vi "GetStatus.vi"(8 "error in (no error)":errorcluster, 11 "S4GUI in":refnum<class "S4GUI.lvclass">) -> (0 "error out":errorcluster, 3 "S4GUI out":refnum<class "S4GUI.lvclass">)   [LabVIEW 2018, in "S4GUI.lvclass"]
uses:
  S4GUI.lvclass
  S4GUI.lvclass/S4GUI.ctl
  Server/Server.lvclass/Server.ctl
  Instrument/Instrument.lvclass/Instrument.ctl
  Device/Optics/Optics.lvclass/Optics.ctl
  Interface/Interface.lvclass/Interface.ctl
  TelFocus/TelFocus.lvclass
  C:/Users/devstaff/sparc4/s4gui/Versao ZeroMQ REQ-REP/SPARC4_GUI -v1.0.0/Server/Server.lvclass
  WeatherStation/WeatherStation.lvclass
  Instrument/Instrument.lvclass
  TCS/TCS.lvclass
  SyncBox/Sync Box.lvclass
  Device/Optics/Opt_Selector/Opt_Selector.lvclass
  C:/Users/devstaff/sparc4/s4gui/Versao ZeroMQ REQ-REP/SPARC4_GUI -v1.0.0/Device/Optics/Optics.lvclass
  Device/Optics/Opt_Continuous/Opt_Continuous.lvclass
  Acquisition/Acquisition.lvclass
  GSserver/GSserver.lvclass
  Channel/Channel.lvclass
  Interface/Interface.lvclass
  GSstatus/GSstatus.lvclass
  SecMirror/SecMirror.lvclass
  WeatherSensor/WeatherSensor.lvclass
  Trigger/Trigger.lvclass
  Device/Optics/Optics.lvclass
  Server/Server.lvclass
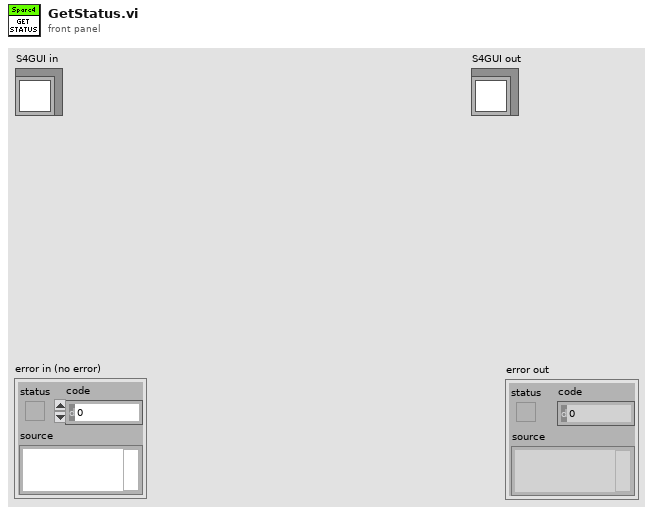
[diagram p1: front panel]
types:
  T1 = cluster{"ACQUISITION_MODE":bool, "TRIGGER_MODE":bool, "READ_MODE":bool, "PREAMP":bool, "READOUT_RATE":bool, "VERTICAL_SHIFT_SPEED":bool, "EM_MODE":bool, "EM_GAIN":bool, "SHUTTER_MODE":bool, "SHUTTER_TTL":bool, "SHUTTER_OPENING_TIME":bool, "SHUTTER_CLOSING_TIME":bool, "VBIN":bool, "HBIN":bool, "INITIAL_LINE":bool, "INITIAL_COLUMN":bool, "FINAL_LINE":bool, "FINAL_COLUMN":bool, "FRAME_TRANSFER":bool, "VERTICAL_CLOCK_VOLTAGE":bool, "AD_CHANNEL":bool}
  T2 = cluster{"ACQUISITION_MODE":u8, "TRIGGER_MODE":u8, "READ_MODE":u8, "PREAMP":u8, "READOUT_RATE":u8, "VERTICAL_SHIFT_SPEED":u8, "EM_MODE":u8, "EM_GAIN":u16, "SHUTTER_MODE":u8, "SHUTTER_TTL":u8, "SHUTTER_OPENING_TIME":u16, "SHUTTER_CLOSING_TIME":u16, "VBIN":u16, "HBIN":u16, "INITIAL_LINE":u16, "INITIAL_COLUMN":u16, "FINAL_LINE":u16, "FINAL_COLUMN":u16, "FRAME_TRANSFER":bool, "VERTICAL_CLOCK_VOLTAGE":u8, "AD_CHANNEL":u32}
  T3 = cluster{"Trigger Mode Status":string, "String output":string, "Instrument Status":cluster{"WPROT pos":dbl, "WPSEL pos":dbl, "GMIR pos":dbl, "GFOC pos":dbl, "CALW pos":dbl, "ASEL pos":dbl, "mode":bool, "String Status":string, "connection":bool, "operational":bool}, "Sync Box State":i32, "Trigger General Status":string, "Instrument States":cluster{"WPSEL State":i32, "WPROT State":i32, "CALW State":i32, "ASEL State":i32, "GMIR State":i32, "GFOC State":i32}, "Instrument Pos Names":cluster{"WPROT posname":string, "WPSEL posname":string, "CALW posname":string, "ASEL posname":string}, "ChannelA_Status":cluster{"Current exp":dbl, "Frames done":u32, "LastFileImage":string, "CamStatus":string, "Run state":u32, "connection":bool, "Cooler ON/OFF":i16, "Currently temperature":i16, "Temperature Status":string, "target  temp":i16, "conf runing":bool, "FT":bool, "UsedDisk":u16, "operational":bool}, "WPROT seq":u16, "ChannelB_Status":cluster{"Current exp":dbl, "Frames done":u32, "LastFileImage":string, "CamStatus":string, "Run state":u32, "connection":bool, "Cooler ON/OFF":i16, "Currently temperature":i16, "Temperature Status":string, "target  temp":i16, "conf runing":bool, "FT":bool, "UsedDisk":u16, "operational":bool}, "ChannelC_Status":cluster{"Current exp":dbl, "Frames done":u32, "LastFileImage":string, "CamStatus":string, "Run state":u32, "connection":bool, "Cooler ON/OFF":i16, "Currently temperature":i16, "Temperature Status":string, "target  temp":i16, "conf runing":bool, "FT":bool, "UsedDisk":u16, "operational":bool}, "ChannelD_Status":cluster{"Current exp":dbl, "Frames done":u32, "LastFileImage":string, "CamStatus":string, "Run state":u32, "connection":bool, "Cooler ON/OFF":i16, "Currently temperature":i16, "Temperature Status":string, "target  temp":i16, "conf runing":bool, "FT":bool, "UsedDisk":u16, "operational":bool}, "ChannelA_CCD":cluster{"ACQUISITION_MODE":u8, "TRIGGER_MODE":u8, "READ_MODE":u8, "PREAMP":u8, "READOUT_RATE":u8, "VERTICAL_SHIFT_SPEED":u8, "EM_MODE":u8, "EM_GAIN":u16, "SHUTTER_MODE":u8, "SHUTTER_TTL":u8, "SHUTTER_OPENNING_TIME":u16, "SHUTTER_CLOSING_TIME":u16, "VBIN":u16, "HBIN":u16, "INITIAL_LINE":u16, "INITIAL_COLUMN":u16, "FINAL_LINE":u16, "FINAL_COLUMN":u16, "FRAME_TRANSFER":bool, "VERTICAL_CLOCK_VOLTAGE":u8, "AD_CHANNEL":u32}, "ChannelB_CCD ":cluster{"ACQUISITION_MODE":u8, "TRIGGER_MODE":u8, "READ_MODE":u8, "PREAMP":u8, "READOUT_RATE":u8, "VERTICAL_SHIFT_SPEED":u8, "EM_MODE":u8, "EM_GAIN":u16, "SHUTTER_MODE":u8, "SHUTTER_TTL":u8, "SHUTTER_OPENNING_TIME":u16, "SHUTTER_CLOSING_TIME":u16, "VBIN":u16, "HBIN":u16, "INITIAL_LINE":u16, "INITIAL_COLUMN":u16, "FINAL_LINE":u16, "FINAL_COLUMN":u16, "FRAME_TRANSFER":bool, "VERTICAL_CLOCK_VOLTAGE":u8, "AD_CHANNEL":u32}, "ChannelC_CCD":cluster{"ACQUISITION_MODE":u8, "TRIGGER_MODE":u8, "READ_MODE":u8, "PREAMP":u8, "READOUT_RATE":u8, "VERTICAL_SHIFT_SPEED":u8, "EM_MODE":u8, "EM_GAIN":u16, "SHUTTER_MODE":u8, "SHUTTER_TTL":u8, "SHUTTER_OPENNING_TIME":u16, "SHUTTER_CLOSING_TIME":u16, "VBIN":u16, "HBIN":u16, "INITIAL_LINE":u16, "INITIAL_COLUMN":u16, "FINAL_LINE":u16, "FINAL_COLUMN":u16, "FRAME_TRANSFER":bool, "VERTICAL_CLOCK_VOLTAGE":u8, "AD_CHANNEL":u32}, "ChannelD_CCD":cluster{"ACQUISITION_MODE":u8, "TRIGGER_MODE":u8, "READ_MODE":u8, "PREAMP":u8, "READOUT_RATE":u8, "VERTICAL_SHIFT_SPEED":u8, "EM_MODE":u8, "EM_GAIN":u16, "SHUTTER_MODE":u8, "SHUTTER_TTL":u8, "SHUTTER_OPENNING_TIME":u16, "SHUTTER_CLOSING_TIME":u16, "VBIN":u16, "HBIN":u16, "INITIAL_LINE":u16, "INITIAL_COLUMN":u16, "FINAL_LINE":u16, "FINAL_COLUMN":u16, "FRAME_TRANSFER":bool, "VERTICAL_CLOCK_VOLTAGE":u8, "AD_CHANNEL":u32}, "CHA_Checked Params":cluster{"ACQUISITION_MODE":bool, "TRIGGER_MODE":bool, "READ_MODE":bool, "PREAMP":bool, "READOUT_RATE":bool, "VERTICAL_SHIFT_SPEED":bool, "EM_MODE":bool, "EM_GAIN":bool, "SHUTTER_MODE":bool, "SHUTTER_TTL":bool, "SHUTTER_OPENING_TIME":bool, "SHUTTER_CLOSING_TIME":bool, "VBIN":bool, "HBIN":bool, "INITIAL_LINE":bool, "INITIAL_COLUMN":bool, "FINAL_LINE":bool, "FINAL_COLUMN":bool, "FRAME_TRANSFER":bool, "VERTICAL_CLOCK_VOLTAGE":bool, "AD_CHANNEL":bool}, "CHB_Checked Params":cluster{"ACQUISITION_MODE":bool, "TRIGGER_MODE":bool, "READ_MODE":bool, "PREAMP":bool, "READOUT_RATE":bool, "VERTICAL_SHIFT_SPEED":bool, "EM_MODE":bool, "EM_GAIN":bool, "SHUTTER_MODE":bool, "SHUTTER_TTL":bool, "SHUTTER_OPENING_TIME":bool, "SHUTTER_CLOSING_TIME":bool, "VBIN":bool, "HBIN":bool, "INITIAL_LINE":bool, "INITIAL_COLUMN":bool, "FINAL_LINE":bool, "FINAL_COLUMN":bool, "FRAME_TRANSFER":bool, "VERTICAL_CLOCK_VOLTAGE":bool, "AD_CHANNEL":bool}, "CHC_Checked Params":cluster{"ACQUISITION_MODE":bool, "TRIGGER_MODE":bool, "READ_MODE":bool, "PREAMP":bool, "READOUT_RATE":bool, "VERTICAL_SHIFT_SPEED":bool, "EM_MODE":bool, "EM_GAIN":bool, "SHUTTER_MODE":bool, "SHUTTER_TTL":bool, "SHUTTER_OPENING_TIME":bool, "SHUTTER_CLOSING_TIME":bool, "VBIN":bool, "HBIN":bool, "INITIAL_LINE":bool, "INITIAL_COLUMN":bool, "FINAL_LINE":bool, "FINAL_COLUMN":bool, "FRAME_TRANSFER":bool, "VERTICAL_CLOCK_VOLTAGE":bool, "AD_CHANNEL":bool}, "CHD_Checked Params":cluster{"ACQUISITION_MODE":bool, "TRIGGER_MODE":bool, "READ_MODE":bool, "PREAMP":bool, "READOUT_RATE":bool, "VERTICAL_SHIFT_SPEED":bool, "EM_MODE":bool, "EM_GAIN":bool, "SHUTTER_MODE":bool, "SHUTTER_TTL":bool, "SHUTTER_OPENING_TIME":bool, "SHUTTER_CLOSING_TIME":bool, "VBIN":bool, "HBIN":bool, "INITIAL_LINE":bool, "INITIAL_COLUMN":bool, "FINAL_LINE":bool, "FINAL_COLUMN":bool, "FRAME_TRANSFER":bool, "VERTICAL_CLOCK_VOLTAGE":bool, "AD_CHANNEL":bool}, "Trigger_connection":bool, "TCSPD_connection":bool, "TCS extended":string, "TCS id":u32, "S4ICS id":u32, "focus pos":i32, "Focus_connection":bool, "WS_connection":bool, "weather status":cluster{"broker":string, "version":string, "date":string, "hour":string, "outHumidity":string, "inHumidity":string, "inTemp":string, "outTemp":string, "windSpeed":string, "windDirection":string, "pressure":string, "dewOut":string, "dewIn":string, "leaf":string, "rain":string, "windChill":string}, "GS STATUS cluster":cluster{"FocusPhot":dbl, "FocusPolar":dbl, "FocusEffic":dbl, "FocusInstrum":dbl, "ICS":bool, "AG":bool, "BROKER":string}, "TCSPD_operational":bool, "Focus_operational":bool}
  T4 = cluster{"TEMP":dbl, "EXPTIME":dbl, "#FRAMES":u32, "#CYCLES":u32, "#SEQS":u32, "WAVEPLATE_POS":u32, "COOLER_POWER_STATUS":dbl, "suffix":string}
  T5 = cluster{"FocusPhot":dbl, "FocusPolar":dbl, "FocusEffic":dbl, "FocusInstrum":dbl, "ICS":bool, "AG":bool, "BROKER":string}
  T6 = cluster{"broker":string, "version":string, "date":string, "hour":string, "outHumidity":string, "intHumidity":string, "inTemp":string, "outTemp":string, "windSpeed":string, "windDirection":string, "pressure":string, "dewOut":string, "dewIn":string, "leaf":string, "rain":string, "windChill":string}
  T7 = cluster{"Texp":dbl, "Nimages":u32, "InitialLine":u32, "FinalLine":u32, "InitialColumn":u32, "FinalColumn":u32, "EmGain":u32, "Cooler Off":bool, "CyclesDone":u32, "SequesDone":u32, "UsedDiskSpace":u16, "Error":bool}
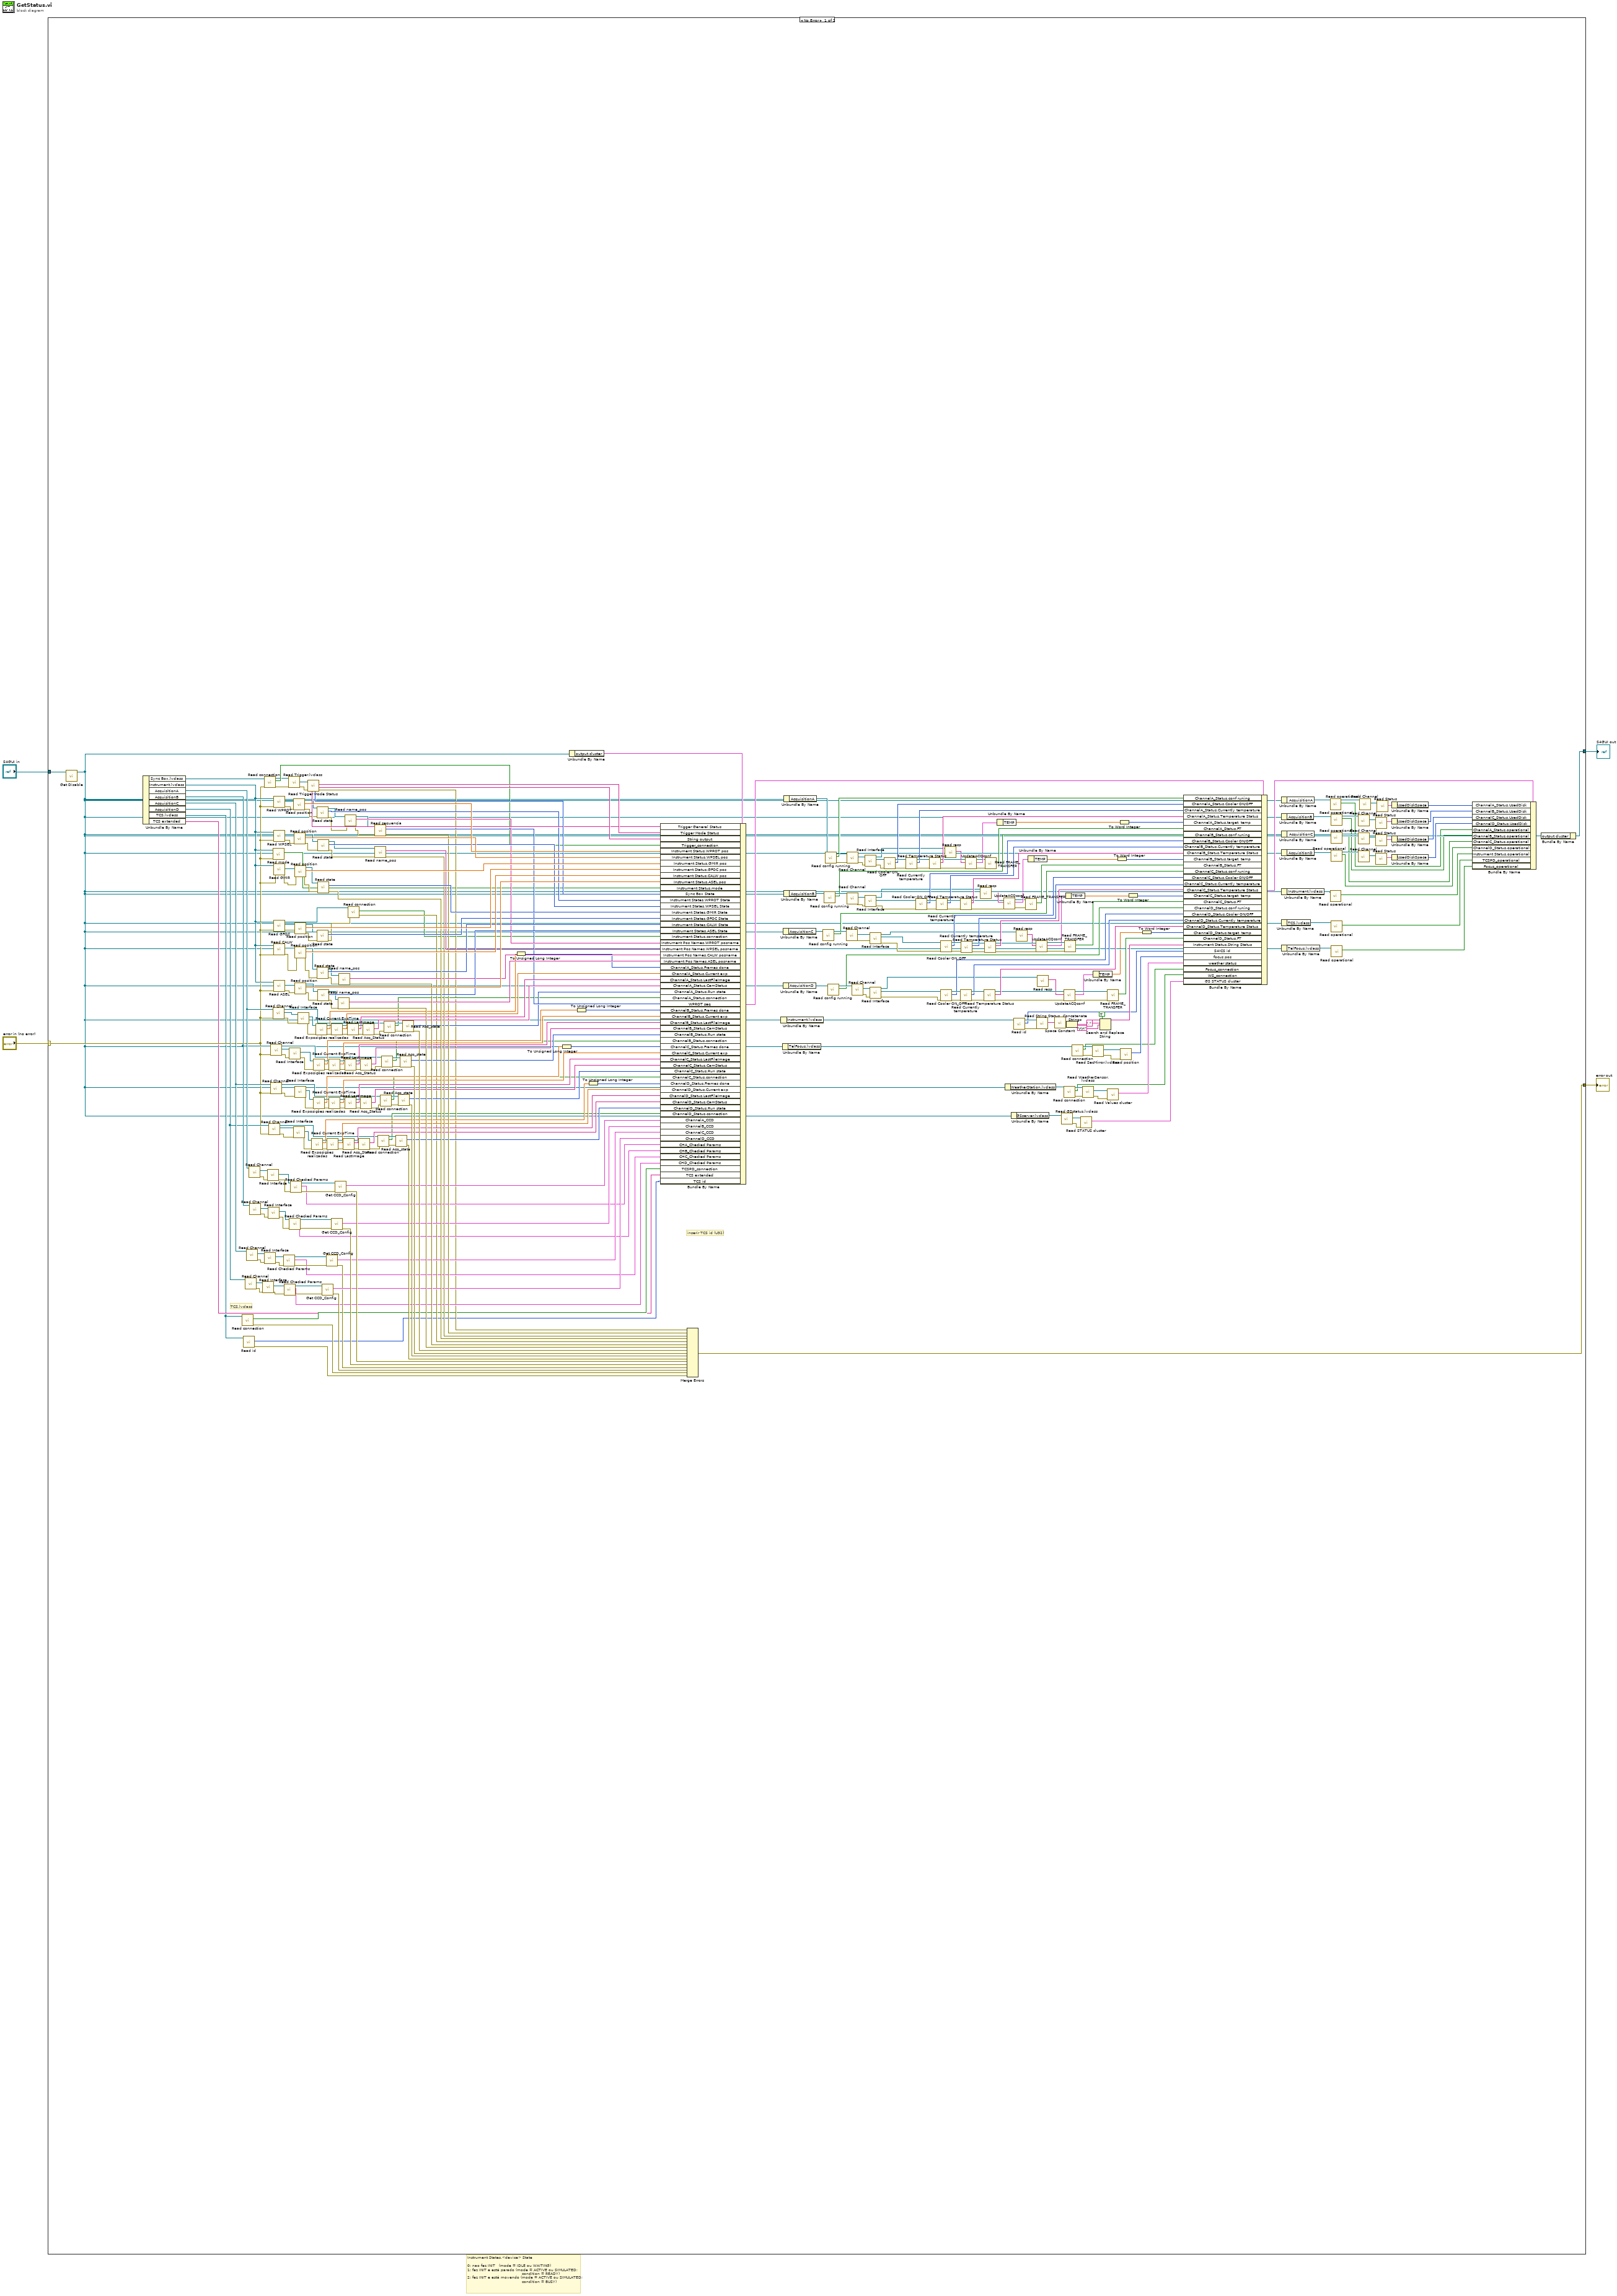
[diagram p0: block diagram]
diagram:
  # "Instrument States.<device> State\n\n0: nao fez INIT   (mode = IDLE ou WAITING)\n1: fez INIT e está parado (mode = ACTIVE ou SIMULATED;\n                                            condition = READY)\n2: fez INIT e está movendo (mode = ACTIVE ou SIMULATED;\n                                            condition = BUSY)"
  n1 = case shown="No Error" "error in (no error)" {
    selector: "error in (no error)" -> [w131 w378]
    tunnel: [w356 w378] -> w3
    tunnel: [w64 w377] -> w1
    tunnel: "S4GUI in" -> [w120 w377]
    frame No Error {
      # "inserir TCS id (U32)"
      # "TCS.lvclass"
      n2 = call-dynamic "Get Disable.vi"("S4ACS_GUI in"=w120) -> ("S4ACS_GUI out"=w60:refnum<class "S4GUI.lvclass">)  [unwired: 9 in, 1 out]
      n3 = Unbundle By Name(w60) -> ("Sync Box.lvclass"=w186:refnum<class "Sync Box.lvclass">, "Instrument.lvclass"=w132:refnum<class "Instrument.lvclass">, "AcquisitionA"=w245:refnum<class "Acquisition.lvclass">, "AcquisitionB"=w240:refnum<class "Acquisition.lvclass">, "AcquisitionC"=w235:refnum<class "Acquisition.lvclass">, "AcquisitionD"=w234:refnum<class "Acquisition.lvclass">, "TCS.lvclass"=w112:refnum<class "TCS.lvclass">, "TCS extended"=w113:string)
      n4 = call "Read connection.vi"("Server in"=w112) -> ("error out"=w110:errorcluster, "connection"=w177:bool)  [unwired: 8 in, 1 out]
      n5 = call "Read id.vi"("Server in"=w112) -> ("error out"=w111:errorcluster, "id"=w109:u32)  [unwired: 8 in, 1 out]
      n6 = call-dynamic "Read Channel.vi"("Acquisition in"=w234) -> ("error out"=w232:errorcluster, "Channel.lvclass"=w233:refnum<class "Channel.lvclass">)  [unwired: 8 in, 1 out]
      n7 = call-dynamic "Read Channel.vi"("Acquisition in"=w235) -> ("error out"=w237:errorcluster, "Channel.lvclass"=w236:refnum<class "Channel.lvclass">)  [unwired: 8 in, 1 out]
      n8 = call-dynamic "Read Channel.vi"("Acquisition in"=w245) -> ("error out"=w246:errorcluster, "Channel.lvclass"=w247:refnum<class "Channel.lvclass">)  [unwired: 8 in, 1 out]
      n9 = call-dynamic "Read Channel.vi"("Acquisition in"=w240) -> ("error out"=w242:errorcluster, "Channel.lvclass"=w241:refnum<class "Channel.lvclass">)  [unwired: 8 in, 1 out]
      n10 = call-dynamic "Read Interface.vi"("error in (no error)"=w232, "Channel in"=w233) -> ("error out"=w214:errorcluster, "Interface.lvclass"=w215:refnum<class "Interface.lvclass">)  [unwired: 7 in, 1 out]
      n11 = call-dynamic "Read Interface.vi"("error in (no error)"=w237, "Channel in"=w236) -> ("error out"=w218:errorcluster, "Interface.lvclass"=w216:refnum<class "Interface.lvclass">)  [unwired: 7 in, 1 out]
      n12 = call "Read connection.vi"("error in (no error)"=w131, "Server in"=w186) -> ("error out"=w183:errorcluster, "connection"=w187:bool, "Server out"=w185:refnum<class "Sync Box.lvclass">)  [unwired: 7 in]
      n13 = call-dynamic "Read Interface.vi"("error in (no error)"=w246, "Channel in"=w247) -> ("error out"=w227:errorcluster, "Interface.lvclass"=w225:refnum<class "Interface.lvclass">)  [unwired: 7 in, 1 out]
      n14 = call-dynamic "Read Interface.vi"("error in (no error)"=w242, "Channel in"=w241) -> ("error out"=w222:errorcluster, "Interface.lvclass"=w220:refnum<class "Interface.lvclass">)  [unwired: 7 in, 1 out]
      n15 = call-dynamic "Read Channel.vi"("error in (no error)"=w131, "Acquisition in"=w234) -> ("error out"=w263:errorcluster, "Channel.lvclass"=w262:refnum<class "Channel.lvclass">, "Acquisition out"=w191:refnum<class "Acquisition.lvclass">)  [unwired: 7 in]
      n16 = call-dynamic "Read Channel.vi"("error in (no error)"=w131, "Acquisition in"=w235) -> ("error out"=w273:errorcluster, "Channel.lvclass"=w272:refnum<class "Channel.lvclass">, "Acquisition out"=w195:refnum<class "Acquisition.lvclass">)  [unwired: 7 in]
      n17 = call-dynamic "Read Channel.vi"("error in (no error)"=w131, "Acquisition in"=w240) -> ("error out"=w290:errorcluster, "Channel.lvclass"=w289:refnum<class "Channel.lvclass">, "Acquisition out"=w199:refnum<class "Acquisition.lvclass">)  [unwired: 7 in]
      n18 = call-dynamic "Read mode.vi"("error in (no error)"=w131, "Instrument in"=w132) -> ("mode"=w130:bool)  [unwired: 7 in, 2 out]
      n19 = call-dynamic "Read Channel.vi"("error in (no error)"=w131, "Acquisition in"=w245) -> ("error out"=w318:errorcluster, "Channel.lvclass"=w319:refnum<class "Channel.lvclass">, "Acquisition out"=w207:refnum<class "Acquisition.lvclass">)  [unwired: 7 in]
      n20 = call "Read WPROT.vi"("error in (no error)"=w131, "Instrument in"=w132) -> ("error out"=w372:errorcluster, "Opt_Selector.lvclass"=w373:refnum<class "Opt_Selector.lvclass">)  [unwired: 7 in, 1 out]
      n21 = call "Read WPSEL.vi"("error in (no error)"=w131, "Instrument in"=w132) -> ("error out"=w374:errorcluster, "Opt_Selector.lvclass"=w371:refnum<class "Opt_Selector.lvclass">)  [unwired: 7 in, 1 out]
      n22 = call "Read GMIR.vi"("error in (no error)"=w131, "Instrument in"=w132) -> ("error out"=w370:errorcluster, "Opt_Continuous.lvclass"=w368:refnum<class "Opt_Continuous.lvclass">)  [unwired: 7 in, 1 out]
      n23 = call "Read GFOC.vi"("error in (no error)"=w131, "Instrument in"=w132) -> ("error out"=w366:errorcluster, "Opt_Continuous.lvclass"=w367:refnum<class "Opt_Continuous.lvclass">, "Instrument out"=w210:refnum<class "Instrument.lvclass">)  [unwired: 7 in]
      n24 = call "Read CALW.vi"("error in (no error)"=w131, "Instrument in"=w132) -> ("error out"=w369:errorcluster, "Opt_Selector.lvclass"=w365:refnum<class "Opt_Selector.lvclass">)  [unwired: 7 in, 1 out]
      n25 = call "Read ASEL.vi"("error in (no error)"=w131, "Instrument in"=w132) -> ("error out"=w364:errorcluster, "Opt_Selector.lvclass"=w363:refnum<class "Opt_Selector.lvclass">)  [unwired: 7 in, 1 out]
      n26 = call "Read Checked Params.vi"("error in (no error)"=w218, "Interface in"=w216) -> ("error out"=w217:errorcluster, "Checked Params"=w201:T1, "Interface out"=w211:refnum<class "Interface.lvclass">)  [unwired: 7 in]
      n27 = call "Read Checked Params.vi"("error in (no error)"=w214, "Interface in"=w215) -> ("error out"=w213:errorcluster, "Checked Params"=w200:T1, "Interface out"=w212:refnum<class "Interface.lvclass">)  [unwired: 7 in]
      n28 = call-dynamic "Read Trigger.lvclass.vi"("error in (no error)"=w183, "Sync Box in"=w185) -> ("error out"=w182:errorcluster, "Trigger.lvclass"=w184:refnum<class "Trigger.lvclass">)  [unwired: 7 in, 1 out]
      n29 = call-dynamic "Read Interface.vi"("error in (no error)"=w290, "Channel in"=w289) -> ("error out"=w295:errorcluster, "Interface.lvclass"=w291:refnum<class "Interface.lvclass">)  [unwired: 7 in, 1 out]
      n30 = call "Read Checked Params.vi"("error in (no error)"=w222, "Interface in"=w220) -> ("error out"=w221:errorcluster, "Checked Params"=w202:T1, "Interface out"=w219:refnum<class "Interface.lvclass">)  [unwired: 7 in]
      n31 = call "Read Checked Params.vi"("error in (no error)"=w227, "Interface in"=w225) -> ("error out"=w226:errorcluster, "Checked Params"=w223:T1, "Interface out"=w224:refnum<class "Interface.lvclass">)  [unwired: 7 in]
      n32 = call-dynamic "Read Interface.vi"("error in (no error)"=w263, "Channel in"=w262) -> ("error out"=w268:errorcluster, "Interface.lvclass"=w264:refnum<class "Interface.lvclass">)  [unwired: 7 in, 1 out]
      n33 = call "Read position.vi"("error in (no error)"=w372, "Optics in"=w373) -> ("error out"=w352:errorcluster, "position"=w362:dbl, "Optics out"=w353:refnum<class "Opt_Selector.lvclass">)  [unwired: 7 in]
      n34 = call "Read position.vi"("error in (no error)"=w374, "Optics in"=w371) -> ("error out"=w349:errorcluster, "position"=w361:dbl, "Optics out"=w350:refnum<class "Opt_Selector.lvclass">)  [unwired: 7 in]
      n35 = call "Read position.vi"("error in (no error)"=w370, "Optics in"=w368) -> ("error out"=w346:errorcluster, "position"=w360:dbl, "Optics out"=w347:refnum<class "Opt_Continuous.lvclass">)  [unwired: 7 in]
      n36 = call "Read position.vi"("error in (no error)"=w366, "Optics in"=w367) -> ("error out"=w342:errorcluster, "position"=w359:dbl, "Optics out"=w343:refnum<class "Opt_Continuous.lvclass">)  [unwired: 7 in]
      n37 = call "Read position.vi"("error in (no error)"=w364, "Optics in"=w363) -> ("error out"=w336:errorcluster, "position"=w357:dbl, "Optics out"=w337:refnum<class "Opt_Selector.lvclass">)  [unwired: 7 in]
      n38 = call "Read position.vi"("error in (no error)"=w369, "Optics in"=w365) -> ("error out"=w339:errorcluster, "position"=w358:dbl, "Optics out"=w340:refnum<class "Opt_Selector.lvclass">)  [unwired: 7 in]
      n39 = call-dynamic "Read Interface.vi"("error in (no error)"=w273, "Channel in"=w272) -> ("error out"=w278:errorcluster, "Interface.lvclass"=w274:refnum<class "Interface.lvclass">)  [unwired: 7 in, 1 out]
      n40 = call-dynamic "Read Interface.vi"("error in (no error)"=w318, "Channel in"=w319) -> ("error out"=w308:errorcluster, "Interface.lvclass"=w317:refnum<class "Interface.lvclass">)  [unwired: 7 in, 1 out]
      n41 = call-dynamic "Read Trigger Mode Status.vi"("error in (no error)"=w182, "Trigger in"=w184) -> ("error out"=w181:errorcluster, "String output"=w375:string, "Trigger Mode Status"=w376:string, "State"=w355:i32, "Trigger General Status"=w354:string)  [unwired: 4 in, 1 out]
      n42 = call-dynamic "Read Exposições realizadas.vi"("error in (no error)"=w268, "Interface in"=w264) -> ("error out"=w269:errorcluster, "Exposições realizadas"=w254:dbl, "Interface out"=w265:refnum<class "Interface.lvclass">)  [unwired: 7 in]
      n43 = call-dynamic "Read Exposições realizadas.vi"("error in (no error)"=w278, "Interface in"=w274) -> ("error out"=w279:errorcluster, "Exposições realizadas"=w261:dbl, "Interface out"=w275:refnum<class "Interface.lvclass">)  [unwired: 7 in]
      n44 = call-dynamic "Read Exposições realizadas.vi"("error in (no error)"=w295, "Interface in"=w291) -> ("error out"=w296:errorcluster, "Exposições realizadas"=w287:dbl, "Interface out"=w292:refnum<class "Interface.lvclass">)  [unwired: 7 in]
      n45 = call-dynamic "Read Exposições realizadas.vi"("error in (no error)"=w308, "Interface in"=w317) -> ("error out"=w307:errorcluster, "Exposições realizadas"=w312:dbl, "Interface out"=w316:refnum<class "Interface.lvclass">)  [unwired: 7 in]
      n46 = call-dynamic "Read state.vi"("error in (no error)"=w352, "Optics in"=w353) -> ("error out"=w334:errorcluster, "state"=w351:u8, "Optics out"=w333:refnum<class "Opt_Selector.lvclass">)  [unwired: 7 in]
      n47 = call-dynamic "Read state.vi"("error in (no error)"=w342, "Optics in"=w343) -> ("error out"=w209:errorcluster, "state"=w341:u8)  [unwired: 7 in, 1 out]
      n48 = call-dynamic "Read state.vi"("error in (no error)"=w339, "Optics in"=w340) -> ("error out"=w327:errorcluster, "state"=w338:u8, "Optics out"=w325:refnum<class "Opt_Selector.lvclass">)  [unwired: 7 in]
      n49 = call-dynamic "Read state.vi"("error in (no error)"=w349, "Optics in"=w350) -> ("error out"=w330:errorcluster, "state"=w348:u8, "Optics out"=w329:refnum<class "Opt_Selector.lvclass">)  [unwired: 7 in]
      n50 = call-dynamic "Read state.vi"("error in (no error)"=w346, "Optics in"=w347) -> ("error out"=w345:errorcluster, "state"=w344:u8)  [unwired: 7 in, 1 out]
      n51 = call-dynamic "Read state.vi"("error in (no error)"=w336, "Optics in"=w337) -> ("error out"=w323:errorcluster, "state"=w335:u8, "Optics out"=w321:refnum<class "Opt_Selector.lvclass">)  [unwired: 7 in]
      n52 = call-dynamic "Get CCD_Config.vi"("error in (no error)"=w213, "Interface in"=w212) -> ("error out"=w228:errorcluster, "output cluster"=w230:T2)  [unwired: 7 in, 1 out]
      n53 = call-dynamic "Get CCD_Config.vi"("error in (no error)"=w217, "Interface in"=w211) -> ("error out"=w229:errorcluster, "output cluster"=w231:T2)  [unwired: 7 in, 1 out]
      n54 = call-dynamic "Read Current ExpTime.vi"("error in (no error)"=w269, "Interface in"=w265) -> ("error out"=w270:errorcluster, "Current ExpTime"=w252:dbl, "Interface out"=w266:refnum<class "Interface.lvclass">)  [unwired: 7 in]
      n55 = call-dynamic "Read Current ExpTime.vi"("error in (no error)"=w279, "Interface in"=w275) -> ("error out"=w280:errorcluster, "Current ExpTime"=w259:dbl, "Interface out"=w276:refnum<class "Interface.lvclass">)  [unwired: 7 in]
      n56 = call-dynamic "Read Current ExpTime.vi"("error in (no error)"=w296, "Interface in"=w292) -> ("error out"=w297:errorcluster, "Current ExpTime"=w285:dbl, "Interface out"=w293:refnum<class "Interface.lvclass">)  [unwired: 7 in]
      n57 = call-dynamic "Read Current ExpTime.vi"("error in (no error)"=w307, "Interface in"=w316) -> ("error out"=w306:errorcluster, "Current ExpTime"=w313:dbl, "Interface out"=w315:refnum<class "Interface.lvclass">)  [unwired: 7 in]
      n58 = call-dynamic "Get CCD_Config.vi"("error in (no error)"=w221, "Interface in"=w219) -> ("error out"=w239:errorcluster, "output cluster"=w238:T2)  [unwired: 7 in, 1 out]
      n59 = call-dynamic "Get CCD_Config.vi"("error in (no error)"=w226, "Interface in"=w224) -> ("error out"=w243:errorcluster, "output cluster"=w244:T2)  [unwired: 7 in, 1 out]
      n60 = call "Read name_pos.vi"("error in (no error)"=w323, "Optics in"=w321) -> ("error out"=w322:errorcluster, "name_pos"=w320:string)  [unwired: 7 in, 1 out]
      n61 = call "Read name_pos.vi"("error in (no error)"=w327, "Optics in"=w325) -> ("error out"=w326:errorcluster, "name_pos"=w324:string)  [unwired: 7 in, 1 out]
      n62 = call-dynamic "Read LastImage.vi"("error in (no error)"=w270, "Interface in"=w266) -> ("error out"=w271:errorcluster, "LastImage"=w251:string, "Interface out"=w267:refnum<class "Interface.lvclass">)  [unwired: 7 in]
      n63 = call-dynamic "Read LastImage.vi"("error in (no error)"=w280, "Interface in"=w276) -> ("error out"=w281:errorcluster, "LastImage"=w258:string, "Interface out"=w277:refnum<class "Interface.lvclass">)  [unwired: 7 in]
      n64 = call "Read name_pos.vi"("error in (no error)"=w334, "Optics in"=w333) -> ("error out"=w303:errorcluster, "name_pos"=w332:string, "Optics out"=w304:refnum<class "Opt_Selector.lvclass">)  [unwired: 7 in]
      n65 = call-dynamic "Read LastImage.vi"("error in (no error)"=w297, "Interface in"=w293) -> ("error out"=w298:errorcluster, "LastImage"=w284:string, "Interface out"=w294:refnum<class "Interface.lvclass">)  [unwired: 7 in]
      n66 = call-dynamic "Read LastImage.vi"("error in (no error)"=w306, "Interface in"=w315) -> ("error out"=w305:errorcluster, "LastImage"=w310:string, "Interface out"=w314:refnum<class "Interface.lvclass">)  [unwired: 7 in]
      n67 = call "Read connection.vi"("error in (no error)"=w209, "Server in"=w210) -> ("error out"=w208:errorcluster, "connection"=w61:bool)  [unwired: 7 in, 1 out]
      n68 = call-dynamic "Read Acq_Status.vi"("error in (no error)"=w271, "Interface in"=w267) -> ("error out"=w190:errorcluster, "Acq_Status"=w250:string)  [unwired: 7 in, 1 out]
      n69 = call-dynamic "Read Acq_Status.vi"("error in (no error)"=w281, "Interface in"=w277) -> ("error out"=w193:errorcluster, "Acq_Status"=w257:string)  [unwired: 7 in, 1 out]
      n70 = call-dynamic "Read Acq_Status.vi"("error in (no error)"=w298, "Interface in"=w294) -> ("error out"=w197:errorcluster, "Acq_Status"=w283:string)  [unwired: 7 in, 1 out]
      n71 = call-dynamic "Read Acq_Status.vi"("error in (no error)"=w305, "Interface in"=w314) -> ("error out"=w205:errorcluster, "Acq_Status"=w309:string)  [unwired: 7 in, 1 out]
      n72 = call-dynamic "Read sequencia.vi"("error in (no error)"=w303, "Opt_Selector in"=w304) -> ("error out"=w302:errorcluster, "sequencia"=w301:u16)  [unwired: 7 in, 1 out]
      n73 = call "Read name_pos.vi"("error in (no error)"=w330, "Optics in"=w329) -> ("error out"=w331:errorcluster, "name_pos"=w328:string)  [unwired: 7 in, 1 out]
      n74 = call "Read connection.vi"("error in (no error)"=w190, "Server in"=w191) -> ("error out"=w189:errorcluster, "connection"=w178:bool, "Server out"=w188:refnum<class "Acquisition.lvclass">)  [unwired: 7 in]
      n75 = call "Read connection.vi"("error in (no error)"=w193, "Server in"=w195) -> ("error out"=w192:errorcluster, "connection"=w179:bool, "Server out"=w194:refnum<class "Acquisition.lvclass">)  [unwired: 7 in]
      n76 = call "Read connection.vi"("error in (no error)"=w197, "Server in"=w199) -> ("error out"=w196:errorcluster, "connection"=w180:bool, "Server out"=w198:refnum<class "Acquisition.lvclass">)  [unwired: 7 in]
      n77 = call "Read connection.vi"("error in (no error)"=w205, "Server in"=w207) -> ("error out"=w204:errorcluster, "connection"=w203:bool, "Server out"=w206:refnum<class "Acquisition.lvclass">)  [unwired: 7 in]
      n78 = call-dynamic "Read Acq_state.vi"("error in (no error)"=w189, "Acquisition in"=w188) -> ("error out"=w248:errorcluster, "Acq_state"=w249:u32)  [unwired: 7 in, 1 out]
      n79 = call-dynamic "Read Acq_state.vi"("error in (no error)"=w192, "Acquisition in"=w194) -> ("error out"=w255:errorcluster, "Acq_state"=w256:u32)  [unwired: 7 in, 1 out]
      n80 = call-dynamic "Read Acq_state.vi"("error in (no error)"=w196, "Acquisition in"=w198) -> ("error out"=w288:errorcluster, "Acq_state"=w282:u32)  [unwired: 7 in, 1 out]
      n81 = call-dynamic "Read Acq_state.vi"("error in (no error)"=w204, "Acquisition in"=w206) -> ("error out"=w299:errorcluster, "Acq_state"=w300:u32)  [unwired: 7 in, 1 out]
      n82 = To Unsigned Long Integer(number=w312) -> (unsigned 32bit integer=w311:u32)
      n83 = To Unsigned Long Integer(number=w261) -> (unsigned 32bit integer=w260:u32)
      n84 = Unbundle By Name(w60) -> ("output cluster"=w63:T3)
      n85 = To Unsigned Long Integer(number=w287) -> (unsigned 32bit integer=w286:u32)
      n86 = To Unsigned Long Integer(number=w254) -> (unsigned 32bit integer=w253:u32)
      n87 = Bundle By Name(cluster=w63, "Trigger General Status"=w354, "Trigger Mode Status"=w376, "String output"=w375, "Trigger_connection"=w187, "Instrument Status.WPROT pos"=w362, "Instrument Status.WPSEL pos"=w361, "Instrument Status.GMIR pos"=w360, "Instrument Status.GFOC pos"=w359, "Instrument Status.CALW pos"=w358, "Instrument Status.ASEL pos"=w357, "Instrument Status.mode"=w130, "Sync Box State"=w355, "Instrument States.WPROT State"=w351, "Instrument States.WPSEL State"=w348, "Instrument States.GMIR State"=w344, "Instrument States.GFOC State"=w341, "Instrument States.CALW State"=w338, "Instrument States.ASEL State"=w335, "Instrument Status.connection"=w61, "Instrument Pos Names.WPROT posname"=w332, "Instrument Pos Names.WPSEL posname"=w328, "Instrument Pos Names.CALW posname"=w324, "Instrument Pos Names.ASEL posname"=w320, "ChannelA_Status.Frames done"=w311, "ChannelA_Status.Current exp"=w313, "ChannelA_Status.LastFileImage"=w310, "ChannelA_Status.CamStatus"=w309, "ChannelA_Status.Run state"=w300, "ChannelA_Status.connection"=w203, "WPROT seq"=w301, "ChannelB_Status.Frames done"=w286, "ChannelB_Status.Current exp"=w285, "ChannelB_Status.LastFileImage"=w284, "ChannelB_Status.CamStatus"=w283, "ChannelB_Status.Run state"=w282, "ChannelB_Status.connection"=w180, "ChannelC_Status.Frames done"=w260, "ChannelC_Status.Current exp"=w259, "ChannelC_Status.LastFileImage"=w258, "ChannelC_Status.CamStatus"=w257, "ChannelC_Status.Run state"=w256, "ChannelC_Status.connection"=w179, "ChannelD_Status.Frames done"=w253, "ChannelD_Status.Current exp"=w252, "ChannelD_Status.LastFileImage"=w251, "ChannelD_Status.CamStatus"=w250, "ChannelD_Status.Run state"=w249, "ChannelD_Status.connection"=w178, "ChannelA_CCD"=w244, "ChannelB_CCD"=w238, "ChannelC_CCD"=w231, "ChannelD_CCD"=w230, "CHA_Checked Params"=w223, "CHB_Checked Params"=w202, "CHC_Checked Params"=w201, "CHD_Checked Params"=w200, "TCSPD_connection"=w177, "TCS extended"=w113, "TCS id"=w109) -> (w62:T3)
      n88 = Merge Errors(w181, w302, w331, w345, w208, w326, w322, w299, w288, w255, w248, w243, w239, w229, w228, w110, w111) -> (w356:errorcluster)
      n89 = Unbundle By Name(w60) -> ("Instrument.lvclass"=w99:refnum<class "Instrument.lvclass">)
      n90 = Unbundle By Name(w60) -> ("TelFocus.lvclass"=w89:refnum<class "TelFocus.lvclass">)
      n91 = Unbundle By Name(w60) -> ("AcquisitionC"=w117:refnum<class "Acquisition.lvclass">)
      n92 = Unbundle By Name(w60) -> ("AcquisitionD"=w115:refnum<class "Acquisition.lvclass">)
      n93 = Unbundle By Name(w60) -> ("AcquisitionA"=w122:refnum<class "Acquisition.lvclass">)
      n94 = Unbundle By Name(w60) -> ("AcquisitionB"=w119:refnum<class "Acquisition.lvclass">)
      n95 = call-dynamic "Read config running.vi"("Server in"=w117) -> ("config running"=w103:bool, "Server out"=w116:refnum<class "Acquisition.lvclass">)  [unwired: 8 in, 1 out]
      n96 = call-dynamic "Read config running.vi"("Server in"=w119) -> ("config running"=w104:bool, "Server out"=w118:refnum<class "Acquisition.lvclass">)  [unwired: 8 in, 1 out]
      n97 = call-dynamic "Read config running.vi"("Server in"=w122) -> ("error out"=w105:errorcluster, "config running"=w106:bool, "Server out"=w121:refnum<class "Acquisition.lvclass">)  [unwired: 8 in]
      n98 = call-dynamic "Read config running.vi"("Server in"=w115) -> ("config running"=w101:bool, "Server out"=w114:refnum<class "Acquisition.lvclass">)  [unwired: 8 in, 1 out]
      n99 = call-dynamic "Read Channel.vi"("Acquisition in"=w116) -> ("error out"=w169:errorcluster, "Channel.lvclass"=w170:refnum<class "Channel.lvclass">)  [unwired: 8 in, 1 out]
      n100 = call-dynamic "Read Channel.vi"("error in (no error)"=w105, "Acquisition in"=w121) -> ("error out"=w175:errorcluster, "Channel.lvclass"=w176:refnum<class "Channel.lvclass">)  [unwired: 7 in, 1 out]
      n101 = call-dynamic "Read Channel.vi"("Acquisition in"=w118) -> ("error out"=w172:errorcluster, "Channel.lvclass"=w173:refnum<class "Channel.lvclass">)  [unwired: 8 in, 1 out]
      n102 = call-dynamic "Read Channel.vi"("Acquisition in"=w114) -> ("error out"=w166:errorcluster, "Channel.lvclass"=w167:refnum<class "Channel.lvclass">)  [unwired: 8 in, 1 out]
      n103 = call-dynamic "Read Interface.vi"("error in (no error)"=w175, "Channel in"=w176) -> ("error out"=w159:errorcluster, "Interface.lvclass"=w174:refnum<class "Interface.lvclass">, "Channel out"=w35:refnum<class "Channel.lvclass">)  [unwired: 7 in]
      n104 = call-dynamic "Read Interface.vi"("error in (no error)"=w172, "Channel in"=w173) -> ("error out"=w153:errorcluster, "Interface.lvclass"=w171:refnum<class "Interface.lvclass">, "Channel out"=w31:refnum<class "Channel.lvclass">)  [unwired: 7 in]
      n105 = call-dynamic "Read Interface.vi"("error in (no error)"=w169, "Channel in"=w170) -> ("error out"=w143:errorcluster, "Interface.lvclass"=w168:refnum<class "Interface.lvclass">, "Channel out"=w17:refnum<class "Channel.lvclass">)  [unwired: 7 in]
      n106 = call-dynamic "Read Interface.vi"("error in (no error)"=w166, "Channel in"=w167) -> ("error out"=w142:errorcluster, "Interface.lvclass"=w165:refnum<class "Interface.lvclass">, "Channel out"=w9:refnum<class "Channel.lvclass">)  [unwired: 7 in]
      n107 = call-dynamic "Read Cooler ON_OFF.vi"("error in (no error)"=w159, "Interface in"=w174) -> ("error out"=w158:errorcluster, "Cooler ON/OFF"=w162:i16, "Interface out"=w164:refnum<class "Interface.lvclass">)  [unwired: 7 in]
      n108 = call-dynamic "Read Currently temperature.vi"("error in (no error)"=w158, "Interface in"=w164) -> ("error out"=w157:errorcluster, "Currently temperature"=w161:i8, "Interface out"=w163:refnum<class "Interface.lvclass">)  [unwired: 7 in]
      n109 = call-dynamic "Read Cooler ON_OFF.vi"("error in (no error)"=w153, "Interface in"=w171) -> ("error out"=w154:errorcluster, "Cooler ON/OFF"=w151:i16, "Interface out"=w152:refnum<class "Interface.lvclass">)  [unwired: 7 in]
      n110 = call-dynamic "Read Temperature Status.vi"("error in (no error)"=w157, "Interface in"=w163) -> ("error out"=w38:errorcluster, "Temperature Status"=w160:string, "Interface out"=w39:refnum<class "Interface.lvclass">)  [unwired: 7 in]
      n111 = call-dynamic "Read Currently temperature.vi"("error in (no error)"=w154, "Interface in"=w152) -> ("error out"=w155:errorcluster, "Currently temperature"=w150:i8, "Interface out"=w156:refnum<class "Interface.lvclass">)  [unwired: 7 in]
      n112 = call-dynamic "Read Cooler ON_OFF.vi"("error in (no error)"=w143, "Interface in"=w168) -> ("error out"=w144:errorcluster, "Cooler ON/OFF"=w138:i16, "Interface out"=w146:refnum<class "Interface.lvclass">)  [unwired: 7 in]
      n113 = call-dynamic "Read Cooler ON_OFF.vi"("error in (no error)"=w142, "Interface in"=w165) -> ("error out"=w141:errorcluster, "Cooler ON/OFF"=w135:i16, "Interface out"=w140:refnum<class "Interface.lvclass">)  [unwired: 7 in]
      n114 = call-dynamic "Read resp.vi"("Device in"=w35) -> ("resp"=w34:string)  [unwired: 8 in, 2 out]
      n115 = call-dynamic "Read Temperature Status.vi"("error in (no error)"=w155, "Interface in"=w156) -> ("error out"=w26:errorcluster, "Temperature Status"=w149:string, "Interface out"=w27:refnum<class "Interface.lvclass">)  [unwired: 7 in]
      n116 = call-dynamic "Read Currently temperature.vi"("error in (no error)"=w141, "Interface in"=w140) -> ("error out"=w147:errorcluster, "Currently temperature"=w134:i8, "Interface out"=w139:refnum<class "Interface.lvclass">)  [unwired: 7 in]
      n117 = call-dynamic "Read Currently temperature.vi"("error in (no error)"=w144, "Interface in"=w146) -> ("error out"=w148:errorcluster, "Currently temperature"=w137:i8, "Interface out"=w145:refnum<class "Interface.lvclass">)  [unwired: 7 in]
      n118 = call-dynamic "UpdateACQconf.vi"("error in (no error)"=w38, "status"=w34, "Interface in"=w39) -> ("error out"=w32:errorcluster, "ACQ conf rx"=w40:T4, "Interface out"=w33:refnum<class "Interface.lvclass">)  [unwired: 6 in]
      n119 = call-dynamic "Read resp.vi"("Device in"=w31) -> ("resp"=w30:string)  [unwired: 8 in, 2 out]
      n120 = call-dynamic "Read Temperature Status.vi"("error in (no error)"=w147, "Interface in"=w139) -> ("error out"=w12:errorcluster, "Temperature Status"=w133:string, "Interface out"=w13:refnum<class "Interface.lvclass">)  [unwired: 7 in]
      n121 = call-dynamic "Read Temperature Status.vi"("error in (no error)"=w148, "Interface in"=w145) -> ("error out"=w19:errorcluster, "Temperature Status"=w136:string, "Interface out"=w21:refnum<class "Interface.lvclass">)  [unwired: 7 in]
      n122 = call-dynamic "Read FRAME_TRANSFER.vi"("error in (no error)"=w32, "Interface in"=w33) -> ("FRAME_TRANSFER"=w108:bool)  [unwired: 7 in, 2 out]
      n123 = Unbundle By Name(w40) -> ("TEMP"=w37:dbl)
      n124 = call-dynamic "UpdateACQconf.vi"("error in (no error)"=w26, "status"=w30, "Interface in"=w27) -> ("error out"=w23:errorcluster, "ACQ conf rx"=w29:T4, "Interface out"=w24:refnum<class "Interface.lvclass">)  [unwired: 6 in]
      n125 = Unbundle By Name(w60) -> ("WeatherStation.lvclass"=w85:refnum<class "WeatherStation.lvclass">)
      n126 = Unbundle By Name(w60) -> ("GSserver.lvclass"=w81:refnum<class "GSserver.lvclass">)
      n127 = call "Read id.vi"("Server in"=w99) -> ("error out"=w96:errorcluster, "id"=w97:u32, "Server out"=w98:refnum<class "Instrument.lvclass">)  [unwired: 8 in]
      n128 = call-dynamic "Read resp.vi"("Device in"=w17) -> ("resp"=w16:string)  [unwired: 8 in, 2 out]
      n129 = call-dynamic "Read FRAME_TRANSFER.vi"("error in (no error)"=w23, "Interface in"=w24) -> ("FRAME_TRANSFER"=w107:bool)  [unwired: 7 in, 2 out]
      n130 = Unbundle By Name(w29) -> ("TEMP"=w28:dbl)
      n131 = call-dynamic "UpdateACQconf.vi"("error in (no error)"=w19, "status"=w16, "Interface in"=w21) -> ("error out"=w18:errorcluster, "ACQ conf rx"=w15:T4, "Interface out"=w20:refnum<class "Interface.lvclass">)  [unwired: 6 in]
      n132 = call-dynamic "Read String Status.vi"("error in (no error)"=w96, "Server in"=w98) -> ("String Status"=w125:string)  [unwired: 7 in, 2 out]
      n133 = call-dynamic "Read resp.vi"("Device in"=w9) -> ("resp"=w8:string)  [unwired: 8 in, 2 out]
      n134 = call <vilib>:"Space Constant.vi"() -> ("String"=w126:string)
      n135 = call-dynamic "Read GSstatus.lvclass.vi"("GSserver in"=w81) -> ("error out"=w79:errorcluster, "GSstatus.lvclass"=w80:refnum<class "GSstatus.lvclass">)  [unwired: 8 in, 1 out]
      n136 = call "Read connection.vi"("Server in"=w85) -> ("error out"=w83:errorcluster, "connection"=w82:bool, "Server out"=w84:refnum<class "WeatherStation.lvclass">)  [unwired: 8 in]
      n137 = call-dynamic "UpdateACQconf.vi"("error in (no error)"=w12, "status"=w8, "Interface in"=w13) -> ("error out"=w10:errorcluster, "ACQ conf rx"=w7:T4, "Interface out"=w11:refnum<class "Interface.lvclass">)  [unwired: 6 in]
      n138 = call-dynamic "Read FRAME_TRANSFER.vi"("error in (no error)"=w18, "Interface in"=w20) -> ("FRAME_TRANSFER"=w102:bool)  [unwired: 7 in, 2 out]
      n139 = Unbundle By Name(w15) -> ("TEMP"=w22:dbl)
      n140 = Concatenate Strings(w126, w125) -> (w124:string)
      n141 = call "Read connection.vi"("Server in"=w89) -> ("error out"=w87:errorcluster, "connection"=w86:bool, "Server out"=w88:refnum<class "TelFocus.lvclass">)  [unwired: 8 in]
      n142 = call-dynamic "Read STATUS cluster.vi"("error in (no error)"=w79, "GSstatus in"=w80) -> ("STATUS cluster"=w78:T5)  [unwired: 7 in, 2 out]
      n143 = call-dynamic "Read WeatherSensor.lvclass.vi"("error in (no error)"=w83, "WeatherStation in"=w84) -> ("error out"=w92:errorcluster, "WeatherSensor.lvclass"=w93:refnum<class "WeatherSensor.lvclass">)  [unwired: 7 in, 1 out]
      n144 = call-dynamic "Read SecMirror.lvclass.vi"("error in (no error)"=w87, "TelFocus in"=w88) -> ("error out"=w94:errorcluster, "SecMirror.lvclass"=w95:refnum<class "SecMirror.lvclass">)  [unwired: 7 in, 1 out]
      n145 = Unbundle By Name(w7) -> ("TEMP"=w6:dbl)
      n146 = Search and Replace String(replace all?=TRUE ("replace all? (F)"), input string=w124, search string=",", replace string="\r\n" ("input string")) -> (result string=w123:string)  [unwired: 4 in, 3 out]
      n147 = call-dynamic "Read FRAME_TRANSFER.vi"("error in (no error)"=w10, "Interface in"=w11) -> ("FRAME_TRANSFER"=w100:bool)  [unwired: 7 in, 2 out]
      n148 = call-dynamic "Read Values cluster.vi"("error in (no error)"=w92, "WeatherSensor in"=w93) -> ("Values cluster"=w90:T6)  [unwired: 7 in, 2 out]
      n149 = To Word Integer(number=w28) -> (16bit integer=w25:i16)
      n150 = To Word Integer(number=w37) -> (16bit integer=w36:i16)
      n151 = call-dynamic "Read position.vi"("error in (no error)"=w94, "SecMirror in"=w95) -> ("position"=w91:i32)  [unwired: 7 in, 2 out]
      n152 = To Word Integer(number=w22) -> (16bit integer=w14:i16)
      n153 = To Word Integer(number=w6) -> (16bit integer=w5:i16)
      n154 = Bundle By Name(cluster=w62, "ChannelA_Status.conf runing"=w106, "ChannelA_Status.Cooler ON/OFF"=w162, "ChannelA_Status.Currently temperature"=w161, "ChannelA_Status.Temperature Status"=w160, "ChannelA_Status.target  temp"=w36, "ChannelA_Status.FT"=w108, "ChannelB_Status.conf runing"=w104, "ChannelB_Status.Cooler ON/OFF"=w151, "ChannelB_Status.Currently temperature"=w150, "ChannelB_Status.Temperature Status"=w149, "ChannelB_Status.target  temp"=w25, "ChannelB_Status.FT"=w107, "ChannelC_Status.conf runing"=w103, "ChannelC_Status.Cooler ON/OFF"=w138, "ChannelC_Status.Currently temperature"=w137, "ChannelC_Status.Temperature Status"=w136, "ChannelC_Status.target  temp"=w14, "ChannelC_Status.FT"=w102, "ChannelD_Status.conf runing"=w101, "ChannelD_Status.Cooler ON/OFF"=w135, "ChannelD_Status.Currently temperature"=w134, "ChannelD_Status.Temperature Status"=w133, "ChannelD_Status.target  temp"=w5, "ChannelD_Status.FT"=w100, "Instrument Status.String Status"=w123, "S4ICS id"=w97, "focus pos"=w91, "weather status"=w90, "Focus_connection"=w86, "WS_connection"=w82, "GS STATUS cluster"=w78) -> (w68:T3)
      n155 = Unbundle By Name(w60) -> ("AcquisitionA"=w59:refnum<class "Acquisition.lvclass">)
      n156 = Unbundle By Name(w60) -> ("AcquisitionB"=w57:refnum<class "Acquisition.lvclass">)
      n157 = Unbundle By Name(w60) -> ("AcquisitionC"=w55:refnum<class "Acquisition.lvclass">)
      n158 = Unbundle By Name(w60) -> ("AcquisitionD"=w53:refnum<class "Acquisition.lvclass">)
      n159 = Unbundle By Name(w60) -> ("Instrument.lvclass"=w51:refnum<class "Instrument.lvclass">)
      n160 = Unbundle By Name(w60) -> ("TCS.lvclass"=w50:refnum<class "TCS.lvclass">)
      n161 = Unbundle By Name(w60) -> ("TelFocus.lvclass"=w49:refnum<class "TelFocus.lvclass">)
      n162 = call-dynamic "Read operational.vi"("Server in"=w59) -> ("operational"=w48:bool, "Server out"=w58:refnum<class "Acquisition.lvclass">)  [unwired: 8 in, 1 out]
      n163 = call-dynamic "Read operational.vi"("Server in"=w51) -> ("operational"=w44:bool)  [unwired: 8 in, 2 out]
      n164 = call-dynamic "Read operational.vi"("Server in"=w57) -> ("operational"=w47:bool, "Server out"=w56:refnum<class "Acquisition.lvclass">)  [unwired: 8 in, 1 out]
      n165 = call-dynamic "Read operational.vi"("Server in"=w55) -> ("operational"=w46:bool, "Server out"=w54:refnum<class "Acquisition.lvclass">)  [unwired: 8 in, 1 out]
      n166 = call-dynamic "Read operational.vi"("Server in"=w53) -> ("operational"=w45:bool, "Server out"=w52:refnum<class "Acquisition.lvclass">)  [unwired: 8 in, 1 out]
      n167 = call-dynamic "Read operational.vi"("Server in"=w50) -> ("operational"=w43:bool)  [unwired: 8 in, 2 out]
      n168 = call-dynamic "Read operational.vi"("Server in"=w49) -> ("operational"=w42:bool)  [unwired: 8 in, 2 out]
      n169 = call-dynamic "Read Channel.vi"("Acquisition in"=w56) -> ("Channel.lvclass"=w74:refnum<class "Channel.lvclass">)  [unwired: 8 in, 2 out]
      n170 = call-dynamic "Read Channel.vi"("Acquisition in"=w54) -> ("Channel.lvclass"=w72:refnum<class "Channel.lvclass">)  [unwired: 8 in, 2 out]
      n171 = call-dynamic "Read Channel.vi"("Acquisition in"=w52) -> ("Channel.lvclass"=w70:refnum<class "Channel.lvclass">)  [unwired: 8 in, 2 out]
      n172 = call-dynamic "Read Channel.vi"("Acquisition in"=w58) -> ("Channel.lvclass"=w77:refnum<class "Channel.lvclass">)  [unwired: 8 in, 2 out]
      n173 = call-dynamic "Read Status.vi"("Channel in"=w74) -> ("Status"=w73:T7)  [unwired: 8 in, 2 out]
      n174 = call-dynamic "Read Status.vi"("Channel in"=w72) -> ("Status"=w71:T7)  [unwired: 8 in, 2 out]
      n175 = call-dynamic "Read Status.vi"("Channel in"=w70) -> ("Status"=w69:T7)  [unwired: 8 in, 2 out]
      n176 = call-dynamic "Read Status.vi"("Channel in"=w77) -> ("Status"=w76:T7)  [unwired: 8 in, 2 out]
      n177 = Unbundle By Name(w76) -> ("UsedDiskSpace"=w75:u16)
      n178 = Unbundle By Name(w73) -> ("UsedDiskSpace"=w67:u16)
      n179 = Unbundle By Name(w71) -> ("UsedDiskSpace"=w66:u16)
      n180 = Unbundle By Name(w69) -> ("UsedDiskSpace"=w65:u16)
      n181 = Bundle By Name(cluster=w68, "ChannelA_Status.UsedDisk"=w75, "ChannelB_Status.UsedDisk"=w67, "ChannelC_Status.UsedDisk"=w66, "ChannelD_Status.UsedDisk"=w65, "ChannelA_Status.operational"=w48, "ChannelB_Status.operational"=w47, "ChannelC_Status.operational"=w46, "ChannelD_Status.operational"=w45, "Instrument Status.operational"=w44, "TCSPD_operational"=w43, "Focus_operational"=w42) -> (w41:T3)
      n182 = Bundle By Name(cluster=w60, "output cluster"=w41) -> (w64:refnum<class "S4GUI.lvclass">)
    }
    frame Error {
    }
  }
  "error out" <- w3
  "S4GUI out" <- w1
